vi "fg_find_key.vi"(10 "key":string[](array[string]), 11 "rows":T1[](array[typedef])) -> (3 "index":i32)   [LabVIEW 2017, in "toml.lvlib"]
uses:
  toml.lvlib
  fg_row.ctl
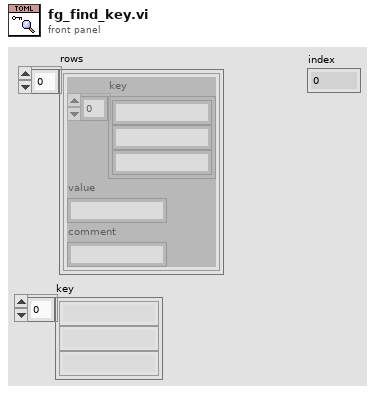
[diagram p1: front panel]
types:
  T1 = typedef "toml.lvlib/fg_row.ctl" = cluster{"key":string[], "value":string, "comment":string}
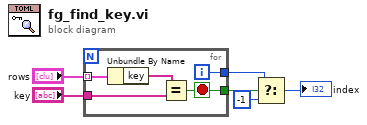
[diagram p0: block diagram]
diagram:
  n1 = for {
    tunnel: "rows" -> [w11] mode=indexing
    tunnel: "key" -> [w9]
    tunnel: [w8] -> w4
    tunnel: [w7] -> w3
    i -> [w8]
    stop <- w7 stop-if-true
    n2 = Unbundle By Name(w11) -> ("key"=w10:string[])
    n3 = Equal?(x=w10, y=w9) -> (x = y?=w7:bool)
  }
  n4 = Select(t=w4, s=w3, f=-1) -> (s? t:f=→"index":i32)
